vi "Login.vi"(8 "error in":errorcluster) -> (0 "error out":errorcluster, 3 "Authentication Service out":refnum<class "Authentication Service.lvclass">)   [LabVIEW 2026, in "Authentication Service.lvclass"]
uses:
  Authentication Service.lvclass
  Authentication Service.lvclass/Authentication Service.ctl
  Interfaces/I Authentication Provider/I Authentication Provider.lvclass
  Domain/Session/Session.lvclass
  Utilities/Time Utils.lvlib
panel:
  out "Session":refnum<class "Session.lvclass">
  in  "Password":string
  in  "Username":string
  in  "Authentication Service in":refnum<class "Authentication Service.lvclass">
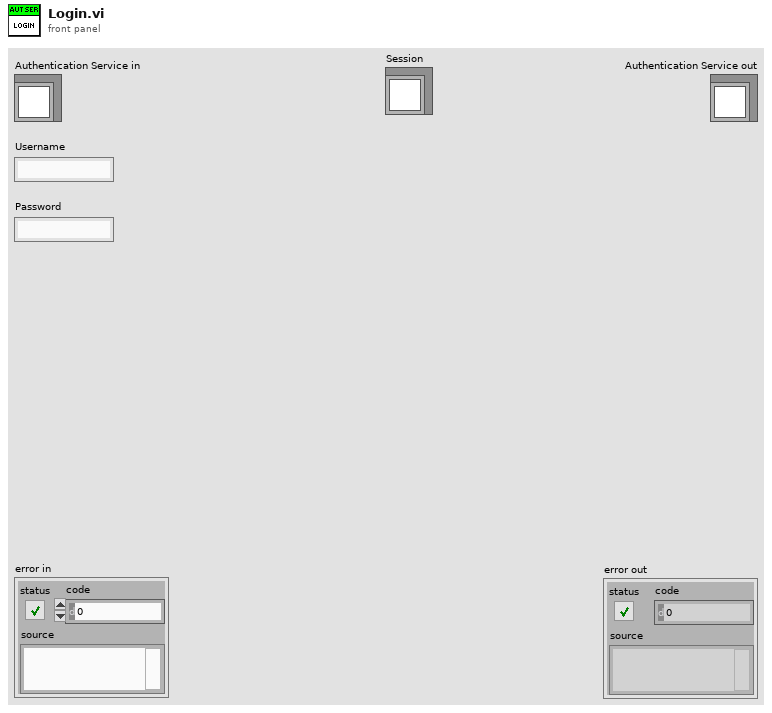
[diagram p1: front panel]
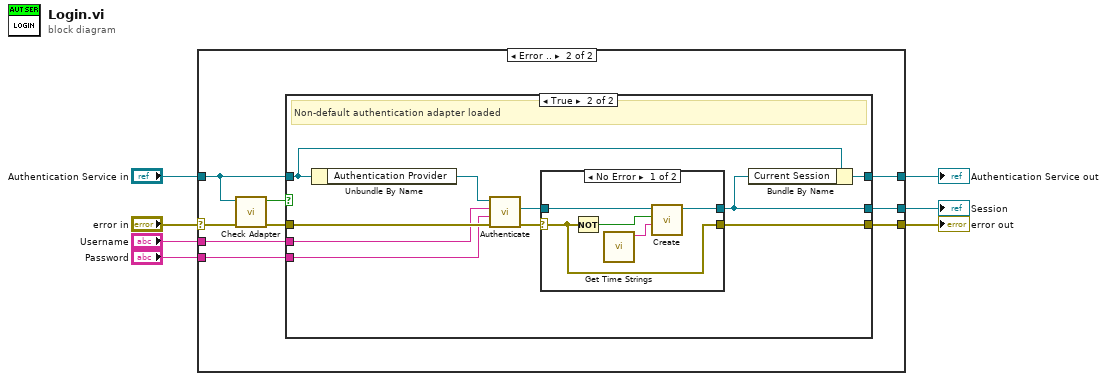
[diagram p0: block diagram]
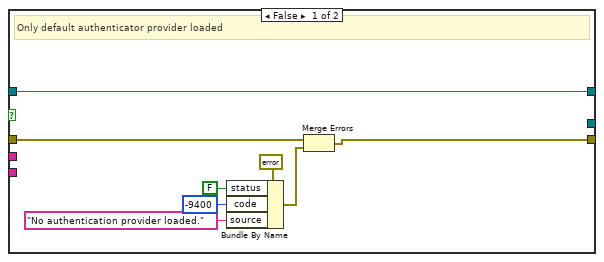
[diagram p3: hidden frame]
diagram:
  n1 = case shown="Error .." "error in" {
    selector: "error in" -> [w9 w18]
    tunnel: [w9 w12] -> w6
    tunnel: "Authentication Service in" -> [w8 w16]
    tunnel: "Username" -> [_ w14]
    tunnel: "Password" -> [_ w13]
    tunnel: [_ w11] -> w2
    tunnel: [w8 w10] -> w1
    frame No Error {
    }
    frame Error {
      n2 = call "Check Adapter.vi"("error in (no error)"=w18, "Authentication Service in"=w16) -> ("error out"=w15:errorcluster, "Adapter Loaded"=w17:bool)  [unwired: 8 in]
      n3 = case shown="True" w17 {
        tunnel: w16 -> [w19 w29]
        tunnel: w15 -> [w22 w35]
        tunnel: w14 -> [_ w34]
        tunnel: w13 -> [_ w33]
        tunnel: [w20 w30] -> w12
        tunnel: [_ w28] -> w11
        tunnel: [w19 w27] -> w10
        frame False {
          # "Only default authenticator provider loaded"
          n4 = Bundle By Name(cluster=errorcluster {"status"=FALSE, "code"=0, "source"=""} ("error IO"), "status"=FALSE, "code"=-9400, "source"="No authentication provider loaded.") -> (w21:errorcluster)
          n5 = Merge Errors(w22, w21) -> (w20:errorcluster)
        }
        frame True {
          # "Non-default authentication adapter loaded"
          n6 = Unbundle By Name(w29) -> ("Authentication Provider"=w36:refnum<class "I Authentication Provider.lvclass">)
          n7 = call-dynamic "Authenticate.vi"("error in (no error)"=w35, "Password"=w33, "Username"=w34, "I Authentication Provider in"=w36) -> ("error out"=w31:errorcluster, "User"=w32:refnum<class "User.lvclass">)  [unwired: 5 in, 1 out]
          n8 = case shown="No Error" w31 {
            selector: w31 -> [w37 w42]
            tunnel: w32 -> [w41 _]
            tunnel: [w38 _] -> w28
            tunnel: [w37 w42] -> w30
            frame No Error {
              n9 = Not(x=w37) -> (.not. x?=w40:bool)
              n10 = call "Get Time Strings.vi"() -> ("YMD HMS with milliseconds"=w39:string)  [unwired: 8 in, 3 out]
              n11 = call "Create.vi"("Start Time"=w39, "Authenticated"=w40, "User"=w41) -> ("Session Data"=w38:refnum<class "Session.lvclass">)  [unwired: 8 in]
            }
            frame Error {
            }
          }
          n12 = Bundle By Name(cluster=w29, "Current Session"=w28) -> (w27:refnum<class "Authentication Service.lvclass">)
        }
      }
    }
  }
  "Authentication Service out" <- w1
  "error out" <- w6
  "Session" <- w2
